vi "Read Selector.vi"(9 "CaseStructure in":refnum<class "CaseStructure.lvclass">) -> (3 "CaseStructure out":refnum<class "CaseStructure.lvclass">, 4 "Selector":refnum<class "Tunnel.lvclass">)   [LabVIEW 2014, in "Raspberry Pi Compatible Compiler for LabVIEW.lvlib" / "CaseStructure.lvclass"]
uses:
  CaseStructure.lvclass
  Tunnel/Tunnel.lvclass
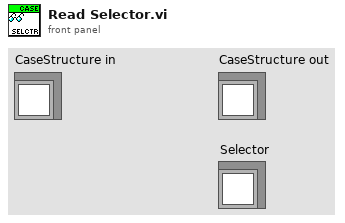
[diagram p1: front panel]
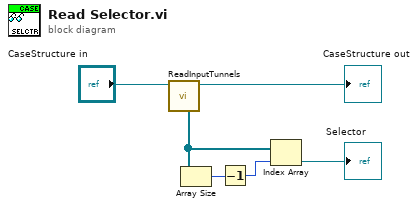
[diagram p0: block diagram]
diagram:
  n1 = call-dynamic "ReadInputTunnels.vi"("Structure in"="CaseStructure in") -> ("Structure out"=→"CaseStructure out":refnum<class "CaseStructure.lvclass">, "tunnels"=w2:refnum<class "Tunnel.lvclass">[])  [unwired: 7 in]
  n2 = Array Size(array=w2) -> (size(s)=w3:i32)
  n3 = Decrement(x=w3) -> (x-1=w1:i32)
  n4 = Index Array(array=w2, index=w1) -> (element=→"Selector":refnum<class "Tunnel.lvclass">)
